vi "Configure Channel (Off) Math.vi"(0 "VISA resource name":refnum<visa-resource-name>, 5 "Math Channel (001)":string="001", 11 "error in (no error)":errorcluster) -> (4 "VISA resource name out":refnum<visa-resource-name>, 6 "Math Channel":string, 15 "error out":errorcluster)   [LabVIEW 2020, in "Yokogawa GX Series.lvlib"]
doc: "Sets the Math channel as off (skip).\n\nCommand: SRangeMath"
uses:
  <instrlib>/Yokogawa GX Series/Yokogawa GX Series.lvlib
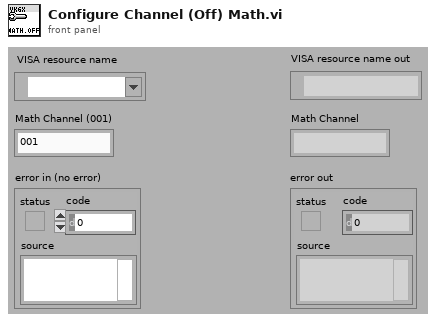
[diagram p1: front panel]
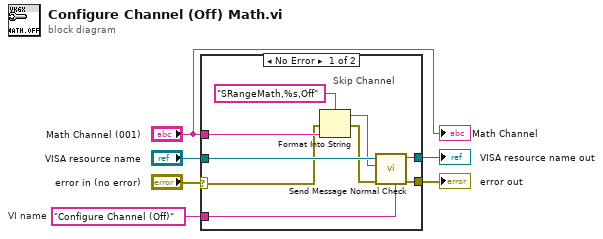
[diagram p0: block diagram]
diagram:
  w5 = "Configure Channel (Off)"  # VI name
  n1 = case shown="No Error" "error in (no error)" {
    selector: "error in (no error)" -> [w7 w16]
    tunnel: "Math Channel (001)" -> [w14 _]
    tunnel: "VISA resource name" -> [w13 w17]
    tunnel: w5 -> [w11 _]
    tunnel: [w9 w17] -> w4
    tunnel: [w8 w16] -> w3
    frame No Error {
      # "Skip Channel"
      n2 = Format Into String(format string="SRangeMath,%s,Off", error in=w7, w14) -> (resulting string=w10:string, error out=w12:errorcluster)  [unwired: 1 in]
      n3 = call <instrlib>:"Send Message Normal Check.vi"("Source (\"\")"=w11, "error in (no error)"=w12, "Send Message (\"\")"=w10, "VISA resource name"=w13) -> ("error out"=w8:errorcluster, "VISA resource name out"=w9:refnum<visa-resource-name>)  [unwired: 1 in, 5 out]
    }
    frame Error {
    }
  }
  "error out" <- w3
  "VISA resource name out" <- w4
  "Math Channel" <- "Math Channel (001)"
